vi "ServoMain.vi"(8 "Error In":errorcluster, 10 "Position in":dbl, 11 "Mode":enum16{"Open", "Control", "Get Value"}(ring)) -> (0 "Error Out":errorcluster, 2 "Position Out":dbl)   [LabVIEW 2016]
uses:
  <vilib>/Rock Robotics/SystemInterfaces/DIO/FPGA_DIOPWMChannel.ctl
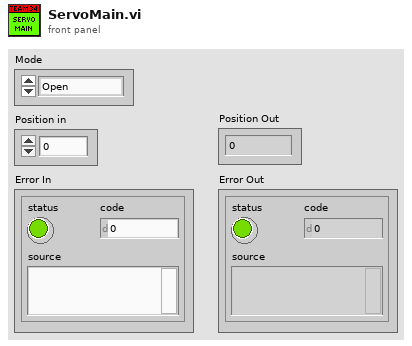
[diagram p1: front panel]
types:
  T1 = typedef "FPGA_DIOPWMChannel.ctl" = enum8{"PWM 0", "PWM 1", "PWM 2", "PWM 3", "PWM 4", "PWM 5", "PWM 6", "PWM 7", "PWM 8", "PWM 9", "PWM MXP 0", "PWM MXP 1", "PWM MXP 2", "PWM MXP 3", "PWM MXP 4", "PWM MXP 5", "PWM MXP 6", "PWM MXP 7", "PWM MXP 8", "PWM MXP 9", "Invalid"}
  T2 = typedef "WPI_ServoDeviceRef.ctl" = cluster{"DeviceStatus":errorcluster, "PWM Channel":T1, "DeadBand":T3}
  T3 = typedef "WPI_PWMDeadband.ctl" = cluster{"Name":string, "maxPositivePwm":i32, "minPositivePwm":i32, "centerPwm":i32, "maxNegativePwm":i32, "minNegativePwm":i32, "angularRange":u16}
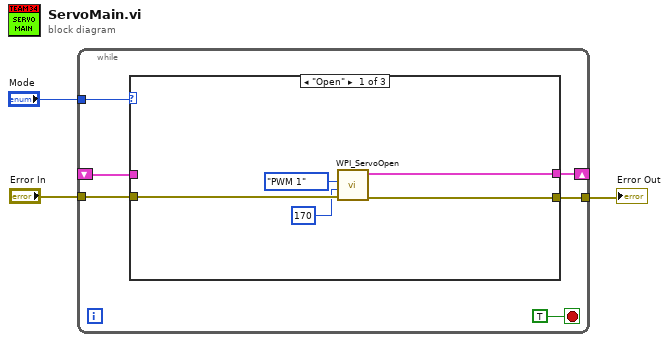
[diagram p0: block diagram]
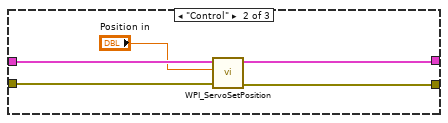
[diagram p2: hidden frame]
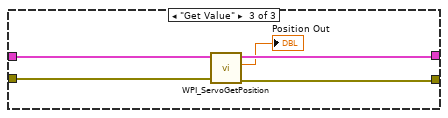
[diagram p3: hidden frame]
diagram:
  n1 = while {
    tunnel: "Mode" -> [w8]
    shift-right: [w7] -> _
    shift-left: _ -> [w6]
    tunnel: "Error In" -> [w5]
    tunnel: [w4] -> w1
    stop <- TRUE stop-if-true
    n2 = case shown="\"Open\"" w8 {
      tunnel: [w14 w19 w23] -> w7
      tunnel: w6 -> [_ w18 w24]
      tunnel: w5 -> [w12 w16 w21]
      tunnel: [w11 w15 w20] -> w4
      frame "Open" {
        n3 = call <vilib>:"WPI_ServoOpen.vi"("error in (no error)"=w12, "Angular Range"=u16 170, "PWM Channel"=FPGA_DIOPWMChannel."PWM 1") -> ("error out"=w11:errorcluster, "ServoDeviceRef"=w14:T2)  [unwired: 7 in]
      }
      frame "Control" {
        n4 = call <vilib>:"WPI_ServoSetPosition.vi"("error in (no error)"=w16, "Position"="Position in", "ServoDeviceRef"=w18) -> ("error out"=w15:errorcluster, "ServoDeviceRef"=w19:T2)  [unwired: 7 in]
      }
      frame "Get Value" {
        n5 = call <vilib>:"WPI_ServoGetPosition.vi"("error in (no error)"=w21, "ServoDeviceRef"=w24) -> ("error out"=w20:errorcluster, "Position"=→"Position Out":dbl, "ServoDeviceRef"=w23:T2)  [unwired: 7 in]
      }
    }
  }
  "Error Out" <- w1
